vi "Begin.vi"(8 "error in":errorcluster) -> (0 "error out":errorcluster)   [LabVIEW 2019]
doc: "Called before other user functions, this VI is expected to open initial I/O refnums, load in file data, and do all program initialization. Notice that the <B>error out</B> terminal is simply used for data flow. Wiring it to other structures or subVIs ensures that this VI runs first."
uses:
  <vilib>/Rock Robotics/WPI/SafetyOutput/WPI_SafetyOutputConfigMenu.ctl
  <vilib>/Rock Robotics/WPI/DriverStation/WPI_DriverStationRobotMode2.ctl
  <vilib>/Rock Robotics/WPI/Joystick/WPI_JoystickDeviceEnum.ctl
  <vilib>/Rock Robotics/WPI/ThirdParty/REV Robotics/SPARK MAX/Typedef/Spark MAX Motor Type.ctl
  <vilib>/Rock Robotics/SystemInterfaces/DIO/FPGA_DIOChannel.ctl
  <vilib>/Rock Robotics/WPI/Solenoid/WPI_SolenoidChannel.ctl
  <vilib>/Rock Robotics/SystemInterfaces/AI/FPGA_AIChannel.ctl
  <vilib>/Rock Robotics/WPI/ThirdParty/Phoenix-LabVIEW/Motor Controller/Controls/CTRE_Phoenix_MotorControl_FeedbackDevice.ctl
  <vilib>/Rock Robotics/SystemInterfaces/i2clib/i2c_bus.ctl
  Robot Global Data.vi
  <vilib>/Rock Robotics/Network Tables/NT Write String Array.vi
  <vilib>/Rock Robotics/WPI/RobotDrive/WPI_RobotDriveOpen4MotorWithExistingMotors.vi
  <vilib>/Rock Robotics/WPI/Switch/WPI_SwitchOpenLimit.vi
  <vilib>/Rock Robotics/WPI/Solenoid/WPI_SolenoidOpenDouble.vi
panel:
  in  "Blue Calibration":cluster{"R":dbl, "G":dbl, "B":dbl}={"R"=0.143, "G"=0.427, "B"=0.429}
  in  "Green Calibration":cluster{"R":dbl, "G":dbl, "B":dbl}={"R"=0.197, "G"=0.561, "B"=0.24}
  in  "Red Calibration":cluster{"R":dbl, "G":dbl, "B":dbl}={"R"=0.561, "G"=0.323, "B"=0.114}
  in  "Yellow Calibration":cluster{"R":dbl, "G":dbl, "B":dbl}={"R"=0.361, "G"=0.524, "B"=0.113}
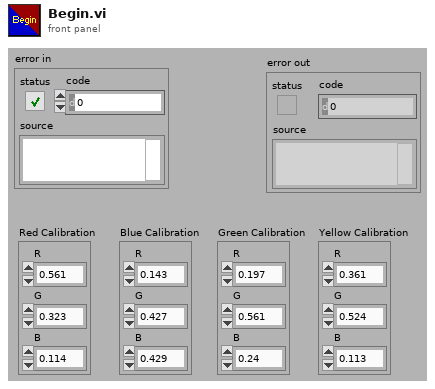
[diagram p1: front panel]
types:
  T1 = typedef "WPI_JoystickDeviceEnum.ctl" = enum16{"USB 0", "USB 1", "USB 2", "USB 3", "USB 4", "USB 5"}
  T2 = typedef "FPGA_DIOChannel.ctl" = enum8{"DIO 0", "DIO 1", "DIO 2", "DIO 3", "DIO 4", "DIO 5", "DIO 6", "DIO 7", "DIO 8", "DIO 9", "DIO MXP 0", "DIO MXP 1", "DIO MXP 2", "DIO MXP 3", "DIO MXP 4", "DIO MXP 5", "DIO MXP 6", "DIO MXP 7", "DIO MXP 8", "DIO MXP 9", "DIO MXP 10", "DIO MXP 11", "DIO MXP 12", "DIO MXP 13", "DIO MXP 14", "DIO MXP 15", "SPI Port CS1", "SPI Port CS2", "SPI Port CS3", "SPI Port MISO", "SPI Port MOSI", "Invalid"}
  T3 = typedef "WPI_SolenoidChannel.ctl" = enum8{"Solenoid 0", "Solenoid 1", "Solenoid 2", "Solenoid 3", "Solenoid 4", "Solenoid 5", "Solenoid 6", "Solenoid 7", "Invalid"}
  T4 = enum16{"FollowerType_PercentOutput", "FollowerType_AuxOutput1"}
  T5 = typedef "CTRE_Phoenix_MotorControl_FeedbackDevice.ctl" = i8
  T6 = typedef "FPGA_AIChannel.ctl" = enum8{"AI 0", "AI 1", "AI 2", "AI 3", "AI MXP 0", "AI MXP 1", "AI MXP 2", "AI MXP 3", "Invalid"}
  T7 = typedef "Spark MAX Motor Type.ctl" = enum16{"Brushed", "Brushless"}
  T8 = typedef "WPI_DriverStationRobotMode2.ctl" = enum16{"Autonomous Disabled", "Autonomous Enabled", "Teleop Disabled", "Teleop Enabled", "Disconnected", "Finish", "Test Disabled", "Test Enabled", "Emergency Stopped"}
  T9 = typedef "WPI_SafetyOutputConfigMenu.ctl" = enum16{"Enable", "Disable"}
  T10 = typedef "WPI_AnalogChannelDevRef.ctl" = cluster{"DevStatus":errorcluster, "Analog Channel":T6}
  T11 = typedef "WPI_DigitalInputDevRef.ctl" = cluster{"DevStatus":errorcluster, "DIO Channel":T2}
  T12 = typedef "WPI_JoystickDevRef.ctl" = cluster{"Device":T1}
  T13 = typedef "WPI_MotorControlDeviceRef.ctl" = cluster{"DeviceStatus":errorcluster, "Type":T14, "PWM":cluster{"PWM Channel":T15, "DeadBand":T16}, "CAN":cluster{"Device Number":u8, "SetOutput VI Ref":variant, "GetOutput VI Ref":variant, "Enable VI Ref":variant, "Disable VI Ref":variant, "Data":variant}, "Invert":bool, "DIO PWM":cluster{"PWM \"Enable\" Channel":T15, "DIOChannel":T2, "PWM Rate":dbl}}
  T14 = typedef "WPI_MotorControlType.ctl" = enum16{"PWM", "CAN", "DIO PWM"}
  T15 = typedef "FPGA_DIOPWMChannel.ctl" = enum8{"PWM 0", "PWM 1", "PWM 2", "PWM 3", "PWM 4", "PWM 5", "PWM 6", "PWM 7", "PWM 8", "PWM 9", "PWM MXP 0", "PWM MXP 1", "PWM MXP 2", "PWM MXP 3", "PWM MXP 4", "PWM MXP 5", "PWM MXP 6", "PWM MXP 7", "PWM MXP 8", "PWM MXP 9", "Invalid"}
  T16 = typedef "WPI_PWMDeadband.ctl" = cluster{"Name":string, "maxPositivePwm":i32, "minPositivePwm":i32, "centerPwm":i32, "maxNegativePwm":i32, "minNegativePwm":i32, "angularRange":u16}
  T17 = typedef "WPI_SolenoidDevRef.ctl" = cluster{"DevStatus":errorcluster, "Pneumatics Control Module":u8, "Forward Solenoid Channel":T3, "Reverse Solenoid Channel":T3}
  T18 = typedef "WPI_RobotDriveDevRef.ctl" = cluster{"DevStatus":errorcluster, "Motors[]":T13[], "Square Inputs":bool, "Max Output":dbl}
  T19 = typedef "WPI_SwitchDevRef.ctl" = cluster{"DevStatus":errorcluster, "DIO Channel":T2, "CntIndex":T20, "Normally Closed":bool}
  T20 = typedef "FPGA_CounterCtrSystemIndex.ctl" = enum8{"Ctr 0", "Ctr 1", "Ctr 2", "Ctr 3", "Ctr 4", "Ctr 5", "Ctr 6", "Ctr 7", "Invalid"}
  T21 = typedef "i2c_bus.ctl" = enum16{"I2C On-Board", "I2C MXP", "Invalid"}
  T22 = typedef "Color Sensor V3 DevRef.ctl" = cluster{"I2CDevRef":T23}
  T23 = typedef "WPI_I2CDevRef.ctl" = cluster{"DevStatus":errorcluster, "Device Address":u8, "Handle":i32, "I2C Bus":T21}
  T24 = typedef "WPI_DigitalOutputDevRef.ctl" = cluster{"DIO Channel":T2, "DevStatus":errorcluster}
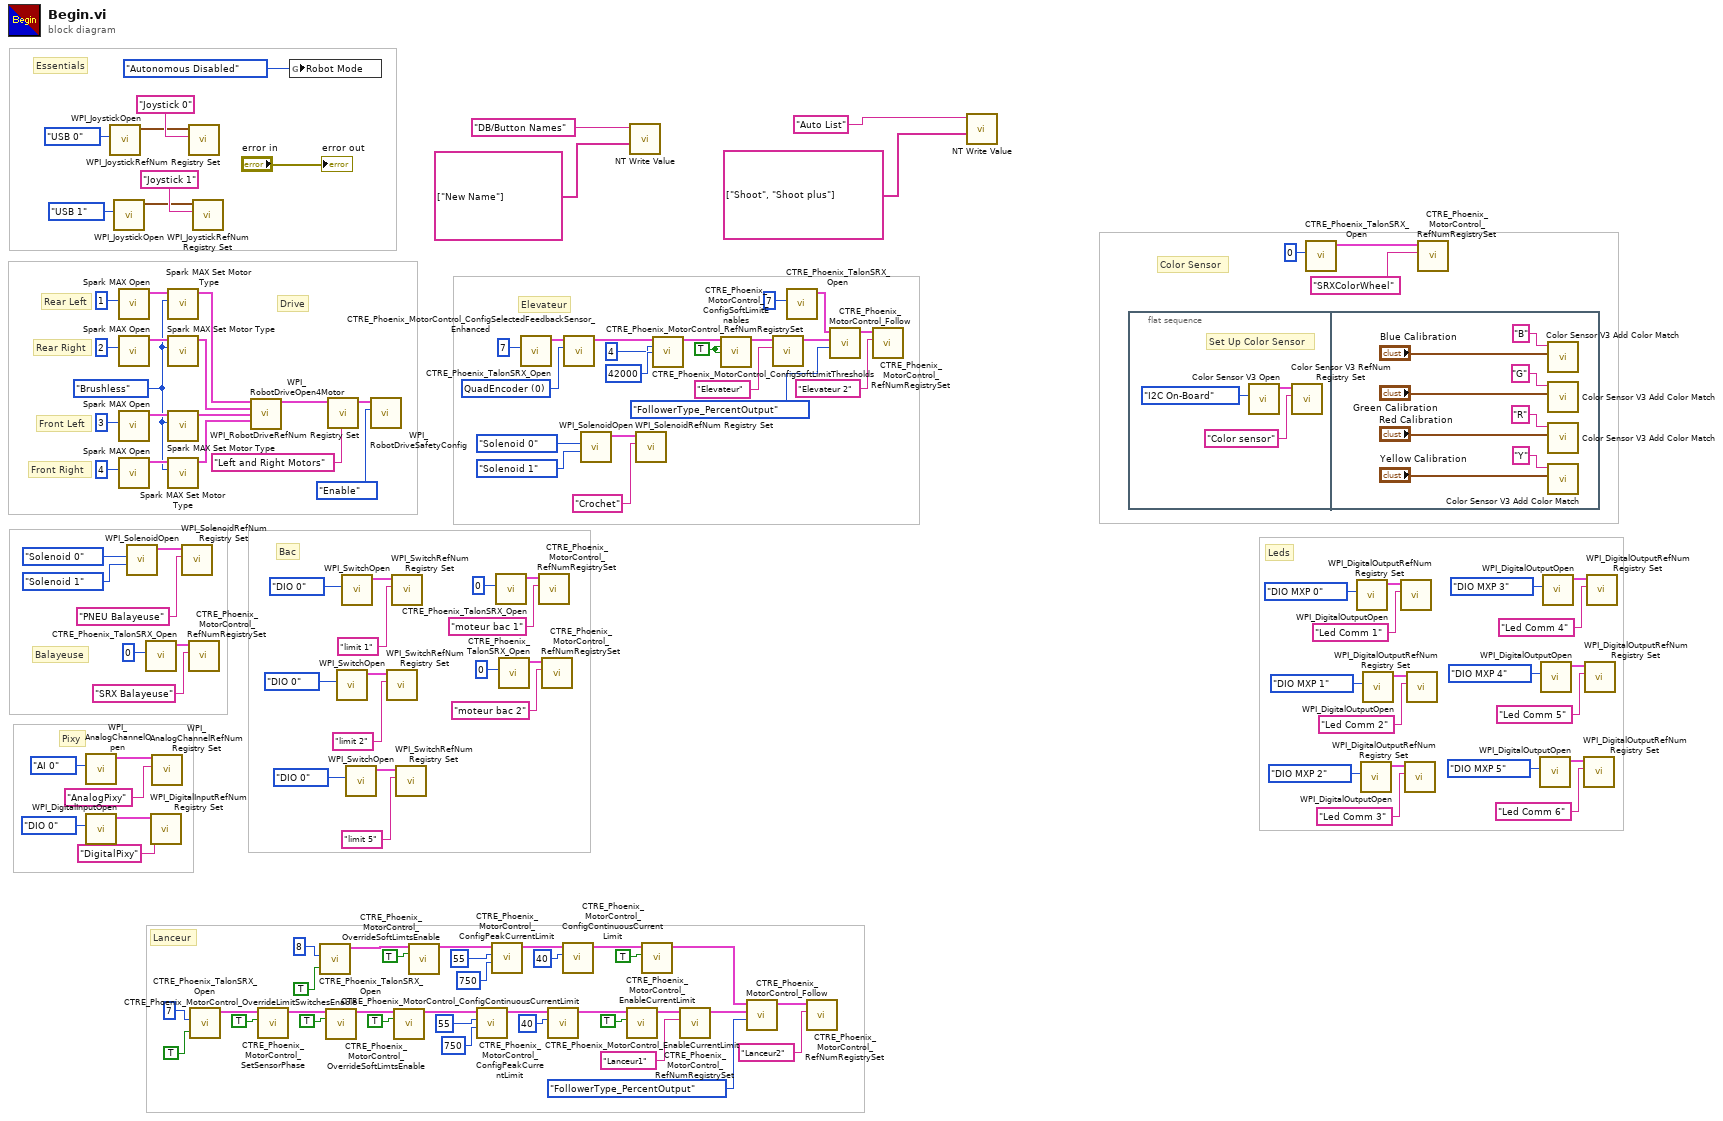
[diagram p0: block diagram]
diagram:
  w40 = TRUE ("Forward Soft Limit Enable")
  w43 = T5 0 items=["None"=-1, "QuadEncoder"=0, "Analog"=2, "Tachometer"=4, "Pulse Width Encoded Position"=8, "Sensor Sum (S0 + S1)"=9, "Sensor Difference (D0 - D1)"=10, "Remote Source 0"=11, "Remote Source 1"=12, "Software Emulated"=15] ("Feedback Device")
  w95 = Spark_MAX_Motor_Type."Brushless" ("Motor Type")
  # "Leds"
  # "Color Sensor"
  # "Elevateur"
  # "Pixy"
  # "Balayeuse"
  # "Bac"
  # "Front Right"
  # "Front Left"
  # "Rear Right"
  # "Rear Left"
  # "Essentials"
  # "Lanceur"
  # "Drive"
  n1 = call <vilib>:"WPI_AnalogChannelOpen.vi"("Analog Channel"=FPGA_AIChannel."AI 0") -> ("AIDeviceRef"=w50:T10)  [unwired: 9 in, 1 out]
  n2 = call <vilib>:"WPI_DigitalInputOpen.vi"("DIO Channel"=FPGA_DIOChannel."DIO 0") -> ("DigitalInputDevRef"=w47:T11)  [unwired: 9 in, 1 out]
  n3 = call <vilib>:"WPI_JoystickOpen.vi"("JoystickDevice"=WPI_JoystickDeviceEnum."USB 0") -> ("JoystickDevRef"=w126:T12)  [unwired: 10 in]
  n4 = call <vilib>:"WPI_JoystickOpen.vi"("JoystickDevice"=WPI_JoystickDeviceEnum."USB 1") -> ("JoystickDevRef"=w2:T12)  [unwired: 10 in]
  n5 = call <vilib>:"Spark MAX Open.vi"("Device Number"=u8 1) -> ("MotorControlDeviceRef"=w106:T13)  [unwired: 9 in, 1 out]
  n6 = call <vilib>:"Spark MAX Open.vi"("Device Number"=u8 2) -> ("MotorControlDeviceRef"=w103:T13)  [unwired: 9 in, 1 out]
  n7 = call <vilib>:"Spark MAX Open.vi"("Device Number"=u8 3) -> ("MotorControlDeviceRef"=w100:T13)  [unwired: 9 in, 1 out]
  n8 = call <vilib>:"Spark MAX Open.vi"("Device Number"=u8 4) -> ("MotorControlDeviceRef"=w97:T13)  [unwired: 9 in, 1 out]
  n9 = call-poly <vilib>:"WPI_SolenoidOpen.vi"("Reverse Solenoid Channel"=WPI_SolenoidChannel."Solenoid 1", "Forward Solenoid Channel"=WPI_SolenoidChannel."Solenoid 0") -> ("SolenoidDevRef"=w57:T17)  [unwired: 8 in, 1 out]
  n10 = call <vilib>:"CTRE_Phoenix_TalonSRX_Open.vi"("Device Number"=u8 0) -> ("CAN Talon SRX Ref"=w54:T13)  [unwired: 9 in, 1 out]
  n11 = call <vilib>:"WPI_DigitalInputRefNum Registry Set.vi"("refnum name"="DigitalPixy", "DigitalInputDevRef"=w47) -> ()  [unwired: 8 in, 2 out]
  n12 = call <vilib>:"WPI_AnalogChannelRefNum Registry Set.vi"("refnum name"="AnalogPixy", "AIDeviceRef"=w50) -> ()  [unwired: 8 in, 2 out]
  n13 = call <vilib>:"Spark MAX Set Motor Type.vi"("Motor Type"=w95, "MotorControlDevRef"=w106) -> ("MotorControlDeviceRef"=w105:T13)  [unwired: 8 in, 1 out]
  n14 = call <vilib>:"Spark MAX Set Motor Type.vi"("Motor Type"=w95, "MotorControlDevRef"=w103) -> ("MotorControlDeviceRef"=w102:T13)  [unwired: 8 in, 1 out]
  n15 = call <vilib>:"Spark MAX Set Motor Type.vi"("Motor Type"=w95, "MotorControlDevRef"=w100) -> ("MotorControlDeviceRef"=w99:T13)  [unwired: 8 in, 1 out]
  n16 = call <vilib>:"Spark MAX Set Motor Type.vi"("Motor Type"=w95, "MotorControlDevRef"=w97) -> ("MotorControlDeviceRef"=w96:T13)  [unwired: 8 in, 1 out]
  n17 = call <vilib>:"WPI_SolenoidRefNum Registry Set.vi"("refnum name"="PNEU Balayeuse", "SolenoidDevRef"=w57) -> ()  [unwired: 8 in, 2 out]
  n18 = call <vilib>:"WPI_JoystickRefNum Registry Set.vi"("refnum name"="Joystick 0", "JoystickDevRef"=w126) -> ()  [unwired: 8 in, 2 out]
  n19 = call <vilib>:"CTRE_Phoenix_MotorControl_RefNumRegistrySet.vi"("refnum name"="SRX Balayeuse", "PhoenixMotorControlDevRef"=w54) -> ()  [unwired: 8 in, 2 out]
  n20 = call <vilib>:"CTRE_Phoenix_TalonSRX_Open.vi"("Invert"=TRUE, "Device Number"=u8 7) -> ("CAN Talon SRX Ref"=w107:T13)  [unwired: 8 in, 1 out]
  n21 = call <vilib>:"WPI_JoystickRefNum Registry Set.vi"("refnum name"="Joystick 1", "JoystickDevRef"=w2) -> ()  [unwired: 8 in, 2 out]
  n22 = call-poly <vilib>:"WPI_RobotDriveOpen4Motor.vi"("Rear Left Motor Dev Ref"=w105, "Rear Right Motor Dev Ref"=w102, "Front Left Motor Dev Ref"=w99, "Front Right Motor Dev Ref"=w96) -> ("RobotDriveDevRef"=w119:T18)  [unwired: 10 in, 1 out]
  n23 = call <vilib>:"CTRE_Phoenix_MotorControl_SetSensorPhase.vi"("PhaseSensor"=TRUE, "PhoenixMotorControlDevRef"=w107) -> ("PhoenixMotorControlDevRef"=w93:T13)  [unwired: 8 in, 1 out]
  n24 = global write "Robot Global Data.vi" "Robot Mode"(WPI_DriverStationRobotMode2."Autonomous Disabled" ("Robot Mode")) -> ()
  n25 = call <vilib>:"CTRE_Phoenix_TalonSRX_Open.vi"("Invert"=TRUE, "Device Number"=u8 8) -> ("CAN Talon SRX Ref"=w74:T13)  [unwired: 8 in, 1 out]
  n26 = call <vilib>:"CTRE_Phoenix_MotorControl_OverrideLimitSwitchesEnable.vi"("PhoenixMotorControlDevRef"=w93, "Override Limit Switch Enable?"=TRUE) -> ("PhoenixMotorControlDevRef"=w94:T13)  [unwired: 12 in, 1 out]
  n27 = call <vilib>:"WPI_RobotDriveRefNum Registry Set.vi"("refnum name"="Left and Right Motors", "RobotDriveDevRef"=w119) -> ("RobotDriveDevRef"=w130:T18)  [unwired: 2 in, 7 out]
  n28 = call-poly <vilib>:"WPI_SwitchOpen.vi"("DIO Channel"=FPGA_DIOChannel."DIO 0") -> ("SwitchDevRef"=w66:T19)  [unwired: 9 in, 1 out]
  n29 = call-poly <vilib>:"WPI_SwitchOpen.vi"("DIO Channel"=FPGA_DIOChannel."DIO 0") -> ("SwitchDevRef"=w64:T19)  [unwired: 9 in, 1 out]
  n30 = call-poly <vilib>:"WPI_SwitchOpen.vi"("DIO Channel"=FPGA_DIOChannel."DIO 0") -> ("SwitchDevRef"=w62:T19)  [unwired: 9 in, 1 out]
  n31 = call <vilib>:"WPI_RobotDriveSafetyConfig.vi"("mode"=WPI_SafetyOutputConfigMenu."Enable", "RobotDriveDevRef"=w130) -> ()  [unwired: 8 in, 2 out]
  n32 = call <vilib>:"WPI_SwitchRefNum Registry Set.vi"("refnum name"="limit 2", "SwitchDevRef"=w66) -> ()  [unwired: 8 in, 2 out]
  n33 = call <vilib>:"WPI_SwitchRefNum Registry Set.vi"("refnum name"="limit 1", "SwitchDevRef"=w64) -> ()  [unwired: 8 in, 2 out]
  n34 = call <vilib>:"CTRE_Phoenix_MotorControl_OverrideSoftLimtsEnable.vi"("PhoenixMotorControlDevRef"=w94, "Override Soft Limit Enable?"=TRUE) -> ("PhoenixMotorControlDevRef"=w90:T13)  [unwired: 12 in, 1 out]
  n35 = call <vilib>:"WPI_SwitchRefNum Registry Set.vi"("refnum name"="limit 5", "SwitchDevRef"=w62) -> ()  [unwired: 8 in, 2 out]
  n36 = call <vilib>:"CTRE_Phoenix_MotorControl_OverrideSoftLimtsEnable.vi"("PhoenixMotorControlDevRef"=w74, "Override Soft Limit Enable?"=TRUE) -> ("PhoenixMotorControlDevRef"=w81:T13)  [unwired: 12 in, 1 out]
  n37 = call <vilib>:"CTRE_Phoenix_MotorControl_ConfigPeakCurrentLimit.vi"("Peak Current Maximum Duration (ms)"=750, "Peak Current (Amps)"=55, "PhoenixMotorControlDevRef"=w90) -> ("PhoenixMotorControlDevRef"=w89:T13)  [unwired: 7 in, 1 out]
  n38 = call <vilib>:"CTRE_Phoenix_MotorControl_ConfigPeakCurrentLimit.vi"("Peak Current Maximum Duration (ms)"=750, "Peak Current (Amps)"=55, "PhoenixMotorControlDevRef"=w81) -> ("PhoenixMotorControlDevRef"=w80:T13)  [unwired: 7 in, 1 out]
  n39 = call <vilib>:"CTRE_Phoenix_TalonSRX_Open.vi"("Device Number"=u8 0) -> ("CAN Talon SRX Ref"=w70:T13)  [unwired: 9 in, 1 out]
  n40 = call <vilib>:"CTRE_Phoenix_TalonSRX_Open.vi"("Device Number"=u8 0) -> ("CAN Talon SRX Ref"=w72:T13)  [unwired: 9 in, 1 out]
  n41 = call <vilib>:"CTRE_Phoenix_TalonSRX_Open.vi"("Device Number"=u8 7) -> ("CAN Talon SRX Ref"=w34:T13)  [unwired: 9 in, 1 out]
  n42 = call <vilib>:"CTRE_Phoenix_MotorControl_RefNumRegistrySet.vi"("refnum name"="moteur bac 1", "PhoenixMotorControlDevRef"=w70) -> ()  [unwired: 8 in, 2 out]
  n43 = call <vilib>:"CTRE_Phoenix_MotorControl_RefNumRegistrySet.vi"("refnum name"="moteur bac 2", "PhoenixMotorControlDevRef"=w72) -> ()  [unwired: 8 in, 2 out]
  n44 = call <vilib>:"CTRE_Phoenix_MotorControl_ConfigContinuousCurrentLimit.vi"("Continuous Current Limit (Amps)"=40, "PhoenixMotorControlDevRef"=w89) -> ("PhoenixMotorControlDevRef"=w88:T13)  [unwired: 8 in, 1 out]
  n45 = call <vilib>:"CTRE_Phoenix_MotorControl_ConfigContinuousCurrentLimit.vi"("Continuous Current Limit (Amps)"=40, "PhoenixMotorControlDevRef"=w80) -> ("PhoenixMotorControlDevRef"=w79:T13)  [unwired: 8 in, 1 out]
  n46 = call <vilib>:"CTRE_Phoenix_MotorControl_ConfigSelectedFeedbackSensor_Enhanced.vi"("Feedback Device"=w43, "PhoenixMotorControlDevRef"=w34) -> ("PhoenixMotorControlDevRef"=w42:T13)  [unwired: 8 in, 1 out]
  n47 = call-poly <vilib>:"WPI_SolenoidOpen.vi"("Reverse Solenoid Channel"=WPI_SolenoidChannel."Solenoid 1", "Forward Solenoid Channel"=WPI_SolenoidChannel."Solenoid 0") -> ("SolenoidDevRef"=w28:T17)  [unwired: 8 in, 1 out]
  n48 = call <vilib>:"CTRE_Phoenix_MotorControl_EnableCurrentLimit.vi"("Enable Current Limit?"=TRUE, "PhoenixMotorControlDevRef"=w88) -> ("PhoenixMotorControlDevRef"=w87:T13)  [unwired: 8 in, 1 out]
  n49 = call-poly <vilib>:"NT Write Value.vi"("String Array"=string[] ["New Name"], "Name"="DB/Button Names") -> ()  [unwired: 9 in, 1 out]
  n50 = call <vilib>:"WPI_SolenoidRefNum Registry Set.vi"("refnum name"="Crochet", "SolenoidDevRef"=w28) -> ()  [unwired: 8 in, 2 out]
  n51 = call <vilib>:"CTRE_Phoenix_MotorControl_EnableCurrentLimit.vi"("Enable Current Limit?"=TRUE, "PhoenixMotorControlDevRef"=w79) -> ("PhoenixMotorControlDevRef"=w73:T13)  [unwired: 8 in, 1 out]
  n52 = call <vilib>:"CTRE_Phoenix_MotorControl_ConfigSoftLimitThresholds.vi"("PhoenixMotorControlDevRef"=w42, "Forward Soft Limit"=4 ("Reverse Soft Limit"), "Reverse Soft Limit"=42000) -> ("PhoenixMotorControlDevRef"=w41:T13)  [unwired: 11 in, 1 out]
  n53 = call <vilib>:"CTRE_Phoenix_MotorControl_RefNumRegistrySet.vi"("refnum name"="Lanceur1", "PhoenixMotorControlDevRef"=w87) -> ("PhoenixMotorControlDevRef"=w109:T13)  [unwired: 8 in, 1 out]
  n54 = call <vilib>:"CTRE_Phoenix_MotorControl_ConfigSoftLimitEnables.vi"("PhoenixMotorControlDevRef"=w41, "Forward Soft Limit Enable"=w40, "Reverse Soft Limit Enable"=w40) -> ("PhoenixMotorControlDevRef"=w33:T13)  [unwired: 11 in, 1 out]
  n55 = call <vilib>:"CTRE_Phoenix_MotorControl_Follow.vi"("FollowerType"=T4."FollowerType_PercentOutput", "Master Controller to Follow"=w109, "PhoenixMotorControlDevRef"=w73) -> ("PhoenixMotorControlDevRef"=w111:T13)  [unwired: 7 in, 1 out]
  n56 = call <vilib>:"CTRE_Phoenix_MotorControl_RefNumRegistrySet.vi"("refnum name"="Elevateur", "PhoenixMotorControlDevRef"=w33) -> ("PhoenixMotorControlDevRef"=w31:T13)  [unwired: 8 in, 1 out]
  n57 = call <vilib>:"CTRE_Phoenix_TalonSRX_Open.vi"("Device Number"=u8 7) -> ("CAN Talon SRX Ref"=w35:T13)  [unwired: 9 in, 1 out]
  n58 = call <vilib>:"CTRE_Phoenix_MotorControl_RefNumRegistrySet.vi"("refnum name"="Lanceur2", "PhoenixMotorControlDevRef"=w111) -> ()  [unwired: 8 in, 2 out]
  n59 = call <vilib>:"CTRE_Phoenix_MotorControl_Follow.vi"("FollowerType"=T4."FollowerType_PercentOutput", "Master Controller to Follow"=w31, "PhoenixMotorControlDevRef"=w35) -> ("PhoenixMotorControlDevRef"=w36:T13)  [unwired: 7 in, 1 out]
  n60 = call <vilib>:"CTRE_Phoenix_MotorControl_RefNumRegistrySet.vi"("refnum name"="Elevateur 2", "PhoenixMotorControlDevRef"=w36) -> ()  [unwired: 8 in, 2 out]
  n61 = call-poly <vilib>:"NT Write Value.vi"("String Array"=string[] ["Shoot", "Shoot plus"], "Name"="Auto List") -> ()  [unwired: 9 in, 1 out]
  n62 = flat-sequence {
    frame #0 {
      # "Set Up Color Sensor"
      n63 = call <vilib>:"Color Sensor V3 Open.vi"("I2C Bus"=i2c_bus."I2C On-Board") -> ("ColorSensorDevRef"=w134:T22)  [unwired: 9 in, 1 out]
      n64 = call <vilib>:"Color Sensor V3 RefNum Registry Set.vi"("refnum name"="Color sensor", "ColorSensorDevRef"=w134) -> ()  [unwired: 8 in, 2 out]
    }
    frame #1 {
      n65 = call <vilib>:"Color Sensor V3 Add Color Match.vi"("Color"="Blue Calibration", "Name"="B") -> ()  [unwired: 10 in]
      n66 = call <vilib>:"Color Sensor V3 Add Color Match.vi"("Color"="Green Calibration", "Name"="G") -> ()  [unwired: 10 in]
      n67 = call <vilib>:"Color Sensor V3 Add Color Match.vi"("Color"="Red Calibration", "Name"="R") -> ()  [unwired: 10 in]
      n68 = call <vilib>:"Color Sensor V3 Add Color Match.vi"("Color"="Yellow Calibration", "Name"="Y") -> ()  [unwired: 10 in]
    }
  }
  n69 = call <vilib>:"CTRE_Phoenix_TalonSRX_Open.vi"("Device Number"=u8 0) -> ("CAN Talon SRX Ref"=w24:T13)  [unwired: 9 in, 1 out]
  n70 = call <vilib>:"WPI_DigitalOutputOpen.vi"("DIO Channel"=FPGA_DIOChannel."DIO MXP 0") -> ("DigitalOutputDevRef"=w21:T24)  [unwired: 9 in, 1 out]
  n71 = call <vilib>:"WPI_DigitalOutputOpen.vi"("DIO Channel"=FPGA_DIOChannel."DIO MXP 2") -> ("DigitalOutputDevRef"=w15:T24)  [unwired: 9 in, 1 out]
  n72 = call <vilib>:"WPI_DigitalOutputOpen.vi"("DIO Channel"=FPGA_DIOChannel."DIO MXP 1") -> ("DigitalOutputDevRef"=w18:T24)  [unwired: 9 in, 1 out]
  n73 = call <vilib>:"WPI_DigitalOutputRefNum Registry Set.vi"("refnum name"="Led Comm 1", "DigitalOutputDevRef"=w21) -> ()  [unwired: 8 in, 2 out]
  n74 = call <vilib>:"WPI_DigitalOutputRefNum Registry Set.vi"("refnum name"="Led Comm 3", "DigitalOutputDevRef"=w15) -> ()  [unwired: 8 in, 2 out]
  n75 = call <vilib>:"WPI_DigitalOutputRefNum Registry Set.vi"("refnum name"="Led Comm 2", "DigitalOutputDevRef"=w18) -> ()  [unwired: 8 in, 2 out]
  n76 = call <vilib>:"CTRE_Phoenix_MotorControl_RefNumRegistrySet.vi"("refnum name"="SRXColorWheel", "PhoenixMotorControlDevRef"=w24) -> ()  [unwired: 8 in, 2 out]
  n77 = call <vilib>:"WPI_DigitalOutputOpen.vi"("DIO Channel"=FPGA_DIOChannel."DIO MXP 5") -> ("DigitalOutputDevRef"=w7:T24)  [unwired: 9 in, 1 out]
  n78 = call <vilib>:"WPI_DigitalOutputOpen.vi"("DIO Channel"=FPGA_DIOChannel."DIO MXP 4") -> ("DigitalOutputDevRef"=w10:T24)  [unwired: 9 in, 1 out]
  n79 = call <vilib>:"WPI_DigitalOutputOpen.vi"("DIO Channel"=FPGA_DIOChannel."DIO MXP 3") -> ("DigitalOutputDevRef"=w12:T24)  [unwired: 9 in, 1 out]
  n80 = call <vilib>:"WPI_DigitalOutputRefNum Registry Set.vi"("refnum name"="Led Comm 6", "DigitalOutputDevRef"=w7) -> ()  [unwired: 8 in, 2 out]
  n81 = call <vilib>:"WPI_DigitalOutputRefNum Registry Set.vi"("refnum name"="Led Comm 5", "DigitalOutputDevRef"=w10) -> ()  [unwired: 8 in, 2 out]
  n82 = call <vilib>:"WPI_DigitalOutputRefNum Registry Set.vi"("refnum name"="Led Comm 4", "DigitalOutputDevRef"=w12) -> ()  [unwired: 8 in, 2 out]
  "error out" <- "error in"
